vi "BRig_RT_comm_webdav_upload__sendData.vi"(8 "input_error":errorcluster, 9 "input_localPath":path, 10 "input_targetPath":string, 11 "input_hSession":T1) -> (0 "error out":errorcluster, 2 "output_sendData":bool, 3 "output_hSession":T1)   [LabVIEW 2014]
uses:
  <vilib>/WebDAVClient/Advanced/SessionHandle.ctl
  <vilib>/WebDAVClient/Advanced/Put File.vi
  <vilib>/WebDAVClient/NI_WebDAV.lvlib
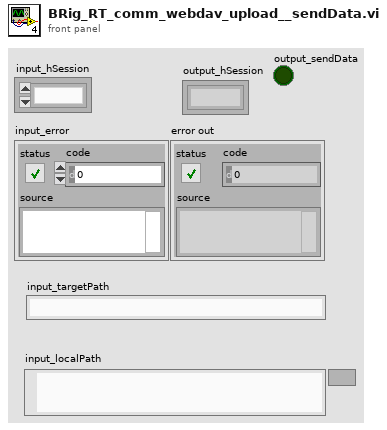
[diagram p1: front panel]
types:
  T1 = typedef "NI_WebDAV.lvlib/SessionHandle.ctl" = refnum<k1>
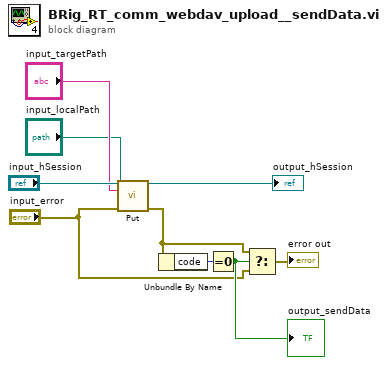
[diagram p0: block diagram]
diagram:
  n1 = call-poly <vilib>:"Put.vi"("session handle"="input_hSession", "relative uri"="input_targetPath", "local file path"="input_localPath", "error in (no error)"="input_error") -> ("session handle out"=→"output_hSession":T1, "error out"=w5:errorcluster)  [unwired: 9 in, 1 out]
  n2 = Unbundle By Name(w5) -> ("code"=w8:i32)
  n3 = Equal To 0?(x=w8) -> (x = 0?=w6:bool)
  "output_sendData" <- w6
  n4 = Select(t=w5, s=w6, f="input_error") -> (s? t:f=→"error out":errorcluster)
